vi "GOOP_GetControlRearrangement.vi"(0 "VI Refnum":refnum<vi>, 1 "_IconSize":u16(ring) caption="Icon Size" items=["Full", "1 c-term high", "2 c-term high", "3 c-term high", "4 c-term high"], 5 "error in (no error)":errorcluster, 7 "ShowIconTerminalNumbers":bool) -> (10 "StartRow":i32, 12 "EndRow":i32, 14 "ControlsToMove":T1(array[cluster]), 15 "LayoutPicture":picture, 16 "ConnectorPaneHeight":i32[](array[numeric]), 18 "NumberOfTerminalAtStart":i32, 19 "error out":errorcluster)   [LabVIEW 2020]
uses:
  <vilib>/Utility/miscctls.llb/LVRectTypeDef.ctl
  <vilib>/Analysis/baseanly.llb/Mean (DBL).vi
  <vilib>/Analysis/NI_AALBase.lvlib
  <resource>/Framework/Providers/Open_GDS/UML/Graphics_class/Graphics.lvclass
panel:
  out "Moved":cluster{"Before":i32, "After":i32}[](array[cluster])
  out "RightUpperSide":cluster{"Left":i16, "TermNo":i32, "Ctrl":bool}[](array[cluster])
  out "LeftUpperSide":cluster{"Left":i16, "TermNo":i32, "Ctrl":bool}[](array[cluster])
  out "DeleteRightSide":cluster{"Top":i16, "TermNo":i32, "Ctrl":bool}[](array[cluster])
  out "DeleteLeftSide":cluster{"Top":i16, "TermNo":i32, "Ctrl":bool}[](array[cluster])
  out "RightSide":cluster{"Top":i16, "TermNo":i32, "Ctrl":bool}[](array[cluster])
  out "LeftSide":cluster{"Top":i16, "TermNo":i32, "Ctrl":bool}[](array[cluster])
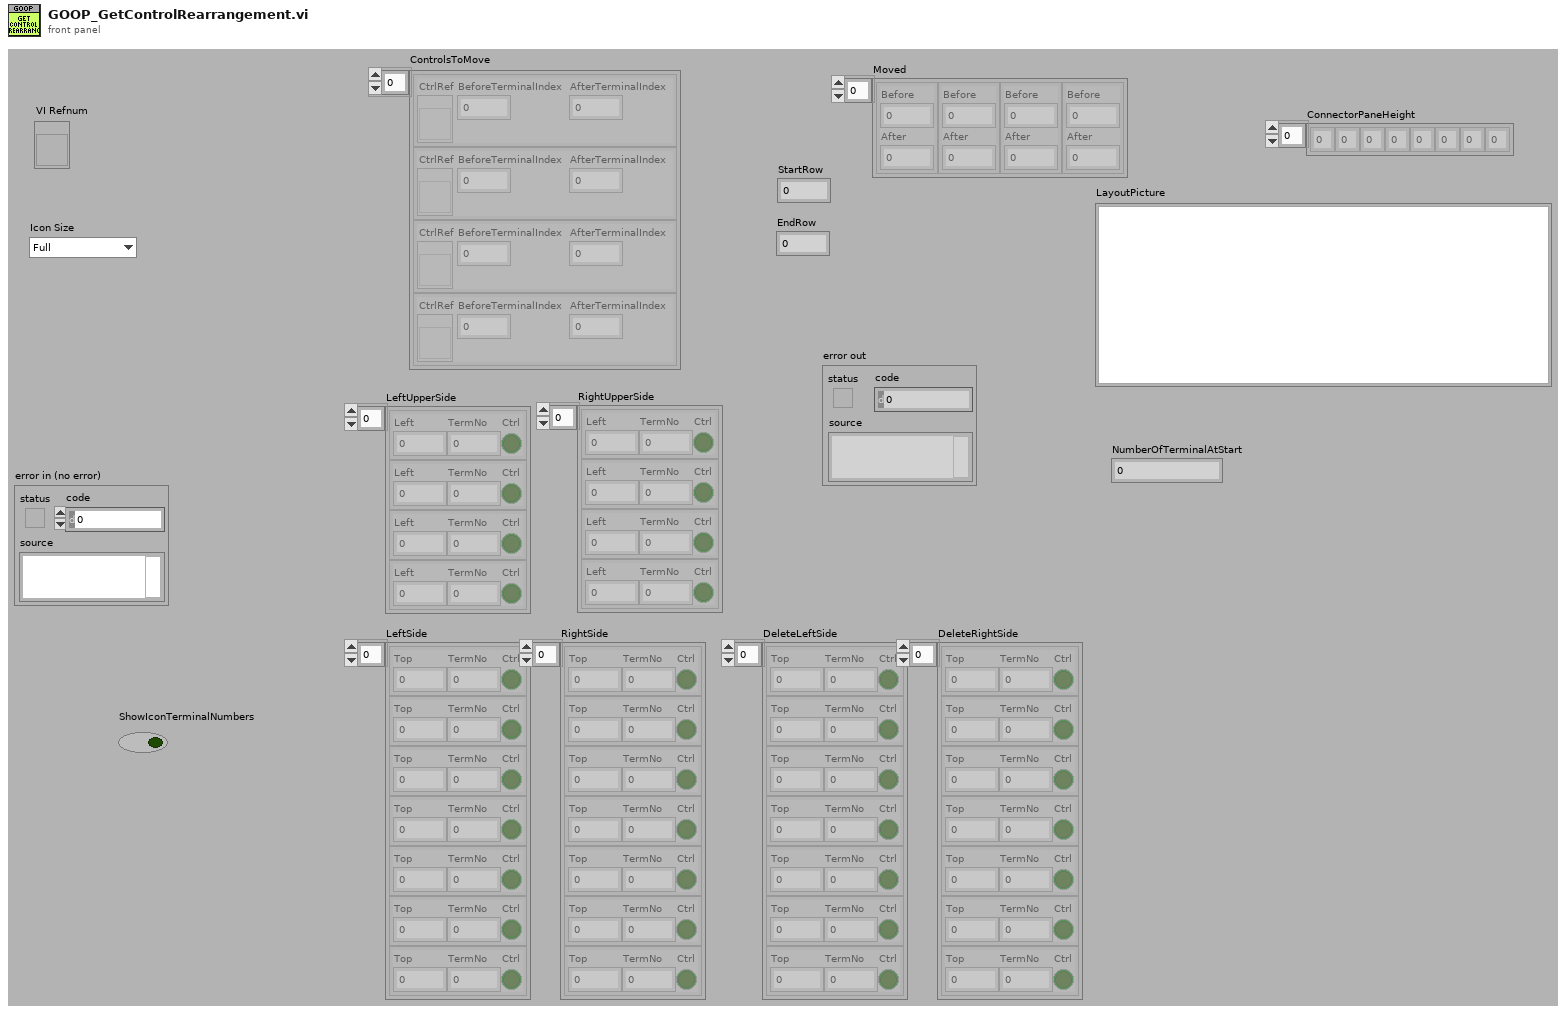
[diagram p1: front panel]
types:
  T1 = cluster{"CtrlRef":refnum<vi>, "BeforeTerminalIndex":i32, "AfterTerminalIndex":i32}[]
  T2 = typedef "LVRectTypeDef.ctl" = cluster{"Left":i16, "Top":i16, "Right":i16, "Bottom":i16}
  T3 = enum32{"invalid VI type", "Standard VI", "Control VI", "Global VI", "Polymorphic VI", "Configuration VI", "SubSystem", "Facade VI", "Method VI", "Statechart Diagram VI"}
  T4 = enum16{"Invalid Wire Rule", "Required", "Recommended", "Optional", "Dynamic Dispatch"}[]
  T5 = typedef "imagedata.ctl" = cluster{"image type":i32, "image depth":i32, "image":u8[], "mask":u8[], "colors":u32[], "Rectangle":cluster{"left":i16, "top":i16, "right":i16, "bottom":i16}}
  T6 = cluster{"horizontal":enum16{"left", "center", "right"}, "vertical":enum16{"top", "center", "bottom"}}
  T7 = enum16{"User-specified Font", "Application Font", "System Font", "Dialog Font"}
  T8 = cluster{"Font Name:":string, "Size":i16, "Strikeout?":bool, "Italic?":bool, "Underline?":bool, "Outline?":bool, "Shadow?":bool, "Bold?":bool}
  T9 = enum16{"Invalid Wire Rule", "Required", "Recommended", "Optional", "Dynamic Dispatch"}
  T10 = cluster{"CtrlRef":refnum<vi>, "BeforeTerminalIndex":i32, "AfterTerminalIndex":i32}
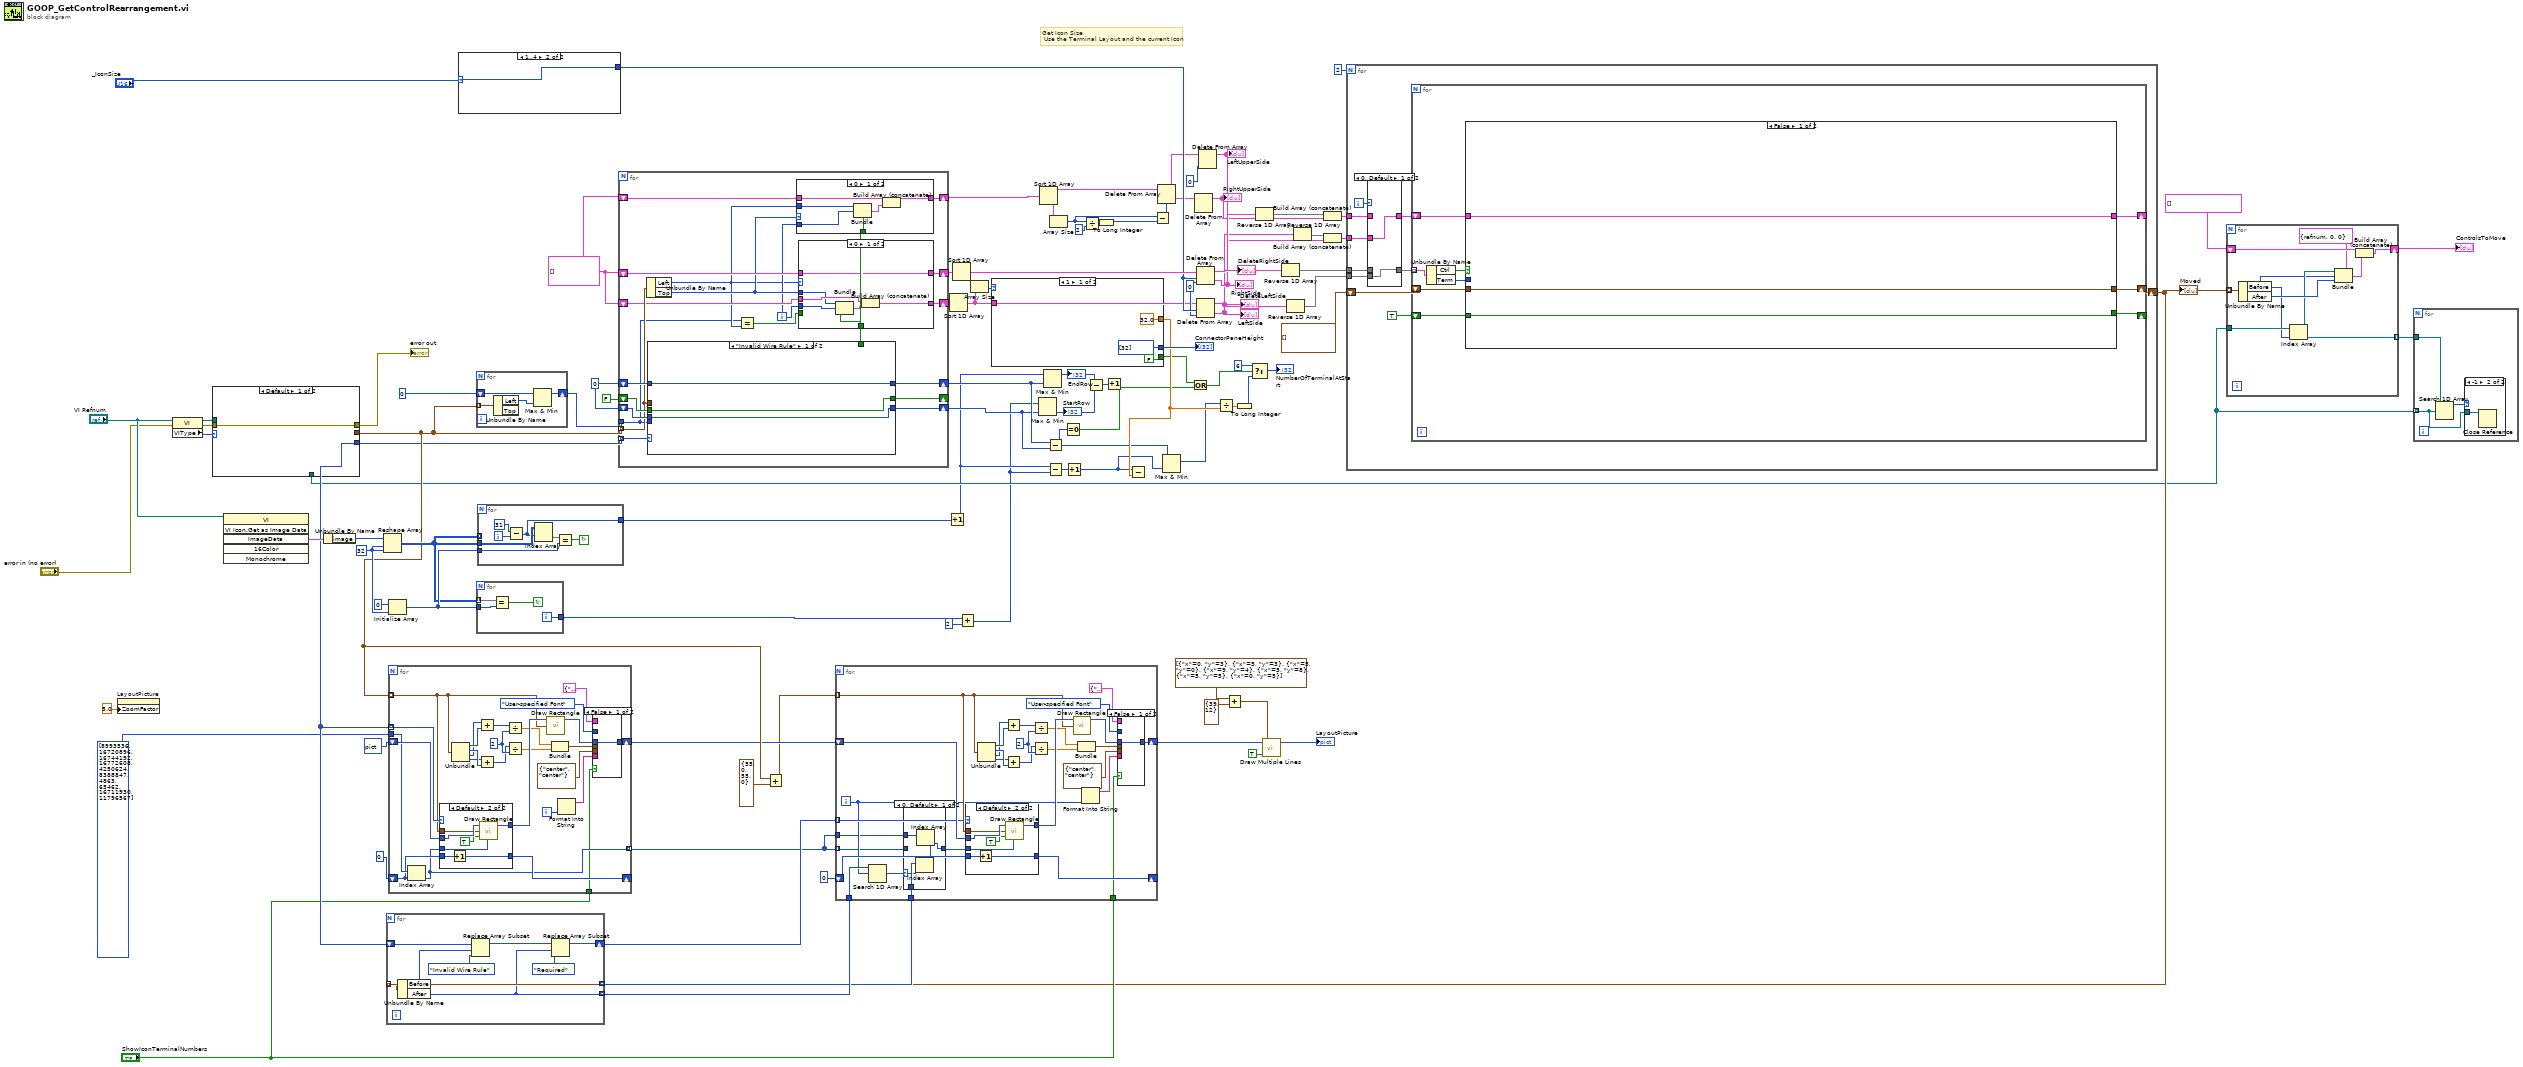
[diagram p0: block diagram]
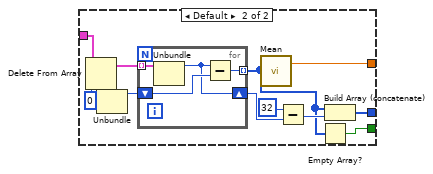
[diagram p2: hidden frame]
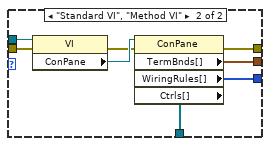
[diagram p3: hidden frame]
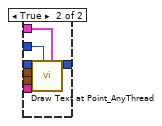
[diagram p5: hidden frame]
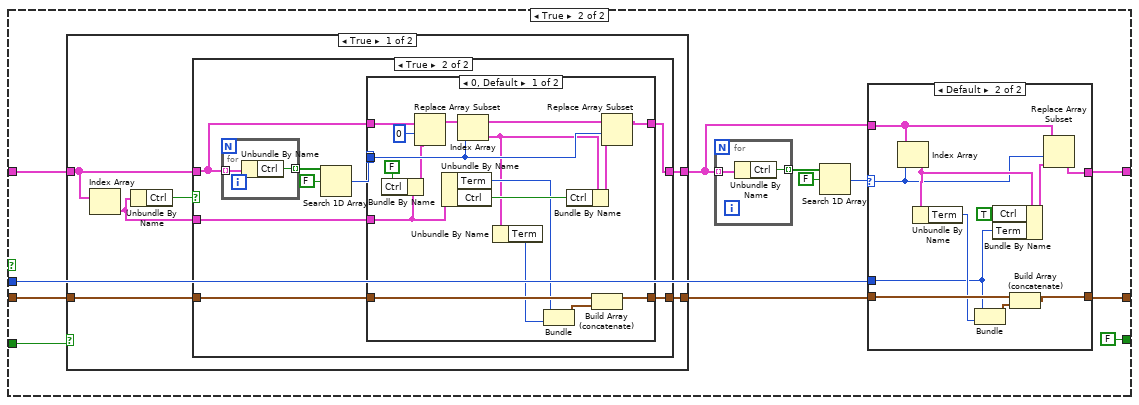
[diagram p9: hidden frame]
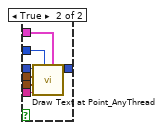
[diagram p14: hidden frame]
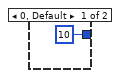
[diagram p16: hidden frame]
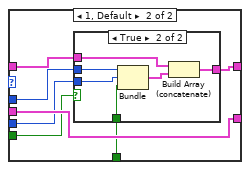
[diagram p18: hidden frame]
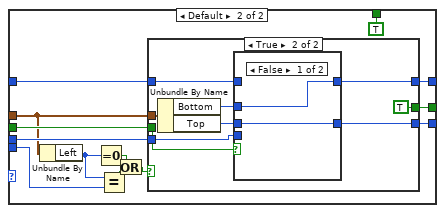
[diagram p20: hidden frame]
diagram:
  w8 = i16 0 ("bottom")
  w83 = 0 ("index")
  w90 = 32 ("dimension size")
  w82 = cluster{"top":i16, "Term":i32, "Ctrl":bool}[] []
  # "Get Icon Size\n Use the Terminal Layout and the current Icon"
  n1 = property on="LayoutPicture" class="Pict"("ZoomFactor"=sgl 5.0 ("Zoom Factor")) -> ()  [unwired: 2 in, 2 out]
  n2 = property class="VI"(reference="VI Refnum", error in="error in (no error)") -> (reference out=w24:refnum<vi>, error out=w23:errorcluster, "VIType"=w21:T3)
  n3 = case shown="Default" w21 {
    tunnel: [_ w105] -> w53
    tunnel: [_ w104] -> w50
    tunnel: [_ w103] -> w33
    tunnel: [w99 w102] -> w31
    tunnel: w24 -> [_ w101]
    tunnel: w23 -> [w99 w100]
    frame Default {
    }
    frame "Standard VI", "Method VI" {
      n4 = property class="VI"(reference=w101, error in=w100) -> (error out=w106:errorcluster, "ConPane"=w107:refnum<vi>)  [unwired: 1 out]
      n5 = property class="ConPane"(reference=w107, error in=w106) -> (error out=w102:errorcluster, "TermBnds[]"=w105:T2[], "WiringRules[]"=w104:T4, "Ctrls[]"=w103:refnum<vi>[])  [unwired: 1 out]
    }
  }
  "error out" <- w31
  n6 = invoke class="VI" method="VI Icon.Get as Image Data"(reference="VI Refnum") -> ("ImageData"=w92:T5)  [unwired: 5 in, 5 out]
  n7 = Unbundle By Name(w92) -> ("image"=w93:u8[])
  n8 = Reshape Array(w93, w90, w90) -> (w88:u8[][])
  n9 = Initialize Array(u8 0 ("element"), w90) -> (w89:u8[])
  n10 = for {
    tunnel: w53 -> [w111] mode=indexing
    shift-right: [w110] -> w52
    shift-left: picture data[5B] ("new picture") -> [w131]
    tunnel: w50 -> [w132] mode=indexing
    tunnel: u32[] [8993536, 16720896, 16744192, 16772608, 4250624, 8388847, 4863, 65462, 16711930, 11796567] -> [w129]
    shift-right: [w127] -> _
    shift-left: 0 -> [w128]
    tunnel: [w109] -> w45 mode=indexing
    tunnel: "ShowIconTerminalNumbers" -> [w108]
    i -> [w133]
    w123 = i16 2 ("y")
    n11 = Index Array(array=w129, index=w128) -> (element=w109:u32)
    n12 = case shown="Default" w132 {
      tunnel: w131 -> [w142 w148]
      tunnel: [w142 w147] -> w130
      tunnel: w111 -> [_ w146]
      tunnel: w128 -> [w143 w150]
      tunnel: [w143 w149] -> w127
      tunnel: w109 -> [_ w144]
      frame "Invalid Wire Rule" {
      }
      frame Default {
        n13 = Increment(x=w150) -> (x+1=w149:i32)
        n14 = call <vilib>:"Draw Rectangle.vi"("picture"=w148, "rect"=w146, "fill?(F)"=TRUE, "color(black)"=w144) -> ("new picture"=w147:picture)  [unwired: 5 in]
      }
    }
    n15 = Unbundle(w111) -> ("Left"=w117:i16, "Top"=w122:i16, "Right"=w116:i16, "Bottom"=w121:i16)
    n16 = Add(x=w116, y=w117) -> (x+y=w118:i16)
    n17 = Add(x=w121, y=w122) -> (x+y=w120:i16)
    n18 = Divide(x=w118, y=w123) -> (x/y=w119:dbl)
    n19 = Divide(x=w120, y=w123) -> (x/y=w124:dbl)
    n20 = call <vilib>:"Draw Rectangle.vi"("picture"=w130, "rect"=w111) -> ("new picture"=w126:picture)  [unwired: 7 in]
    n21 = Bundle(w119, w124) -> (w115:cluster{dbl, dbl})  [unwired: 1 in]
    n22 = Format Into String(w133) -> (resulting string=w125:string)  [unwired: 3 in, 1 out]
    n23 = case shown="False" w108 {
      tunnel: w126 -> [w134 w141]
      tunnel: w125 -> [_ w140]
      tunnel: w115 -> [_ w139]
      tunnel: T6 {"horizontal"=enum."center", "vertical"=enum."center"} ("alignment(left, top)") -> [_ w138]
      tunnel: T8 {"Font Name:"="Arial", "Size"=8, "Strikeout?"=FALSE, "Italic?"=FALSE, "Underline?"=FALSE, "Outline?"=FALSE, "Shadow?"=FALSE, "Bold?"=FALSE} ("[user-specified font]") -> [_ w137]
      tunnel: T7."User-specified Font" ("desired font(Application)") -> [_ w136]
      tunnel: [w134 w135] -> w110
      frame False {
      }
      frame True {
        n24 = call <resource>:"Draw Text at Point_AnyThread.vi"("[user-specified font]"=w137, "desired font(Application)"=w136, "text"=w140, "alignment(left, top)"=w138, "origin"=w139, "picture"=w141) -> ("new picture"=w135:picture)  [unwired: 4 in, 1 out]
      }
    }
  }
  n25 = case shown="1..4" "_IconSize" {
    selector: "_IconSize" -> [_ w152]
    tunnel: [10 w152] -> w84
    frame 0, Default {
    }
    frame 1..4 {
    }
  }
  n26 = for {
    tunnel: w53 -> [w156] mode=indexing
    shift-right: [w153] -> w95
    shift-left: i16 0 -> [w154]
    n27 = Unbundle By Name(w156) -> ("Left"=w155:i16)  [unwired: 1 out]
    n28 = Max & Min(x=w154, y=w155) -> (max(x,y)=w153:i16)  [unwired: 1 out]
  }
  n29 = for {
    tunnel: w88 -> [w160] mode=indexing
    tunnel: w89 -> [w159]
    tunnel: [w157] -> w20
    i -> [w157]
    stop <- w158 continue-if-true
    n30 = Equal?(x=w160, y=w159) -> (x = y?=w158:bool)
  }
  n31 = for {
    tunnel: w88 -> [_] mode=indexing
    tunnel: w89 -> [w167]
    tunnel: w88 -> [w165]
    tunnel: [w161] -> w87
    i -> [w164]
    stop <- w166 continue-if-true
    n32 = Subtract(x=31, y=w164) -> (x-y=w161:i32)
    n33 = Index Array(array=w165, index (row)=w161) -> (element=w162:u8[])  [unwired: 1 in]
    n34 = Equal?(x=w162, y=w167) -> (x = y?=w166:bool)
  }
  n35 = for {
    tunnel: w50 -> [w187] mode=indexing
    tunnel: w53 -> [w180] mode=indexing
    shift-right: [w186] -> w18
    shift-left: w8 -> [w184]
    shift-right: [w185] -> w17
    shift-left: w8 -> [w183]
    shift-right: [w181] -> _
    shift-left: FALSE -> [w182]
    shift-right: [w179] -> w97
    shift-left: w82 -> [w178]
    tunnel: w95 -> [w168]
    shift-right: [w175] -> w94
    shift-left: w82 -> [w176]
    shift-right: [w172] -> w81
    shift-left: w82 -> [w173]
    i -> [w171]
    n36 = Unbundle By Name(w180) -> ("Left"=w170:i16, "Top"=w174:i16)
    n37 = case shown="\"Invalid Wire Rule\"" w187 {
      tunnel: w180 -> [_ w224]
      tunnel: w182 -> [w216 w231]
      tunnel: [w218 w230] -> w186
      tunnel: [w217 w229] -> w185
      tunnel: w184 -> [w218 w228]
      tunnel: w183 -> [w217 w227]
      tunnel: [w216 w226] -> w181
      tunnel: [_ TRUE] -> w169
      tunnel: w168 -> [_ w222]
      frame "Invalid Wire Rule" {
      }
      frame Default {
        n38 = Unbundle By Name(w224) -> ("Left"=w223:i16)
        n39 = Equal To 0?(x=w223) -> (x = 0?=w221:bool)
        n40 = Equal?(x=w223, y=w222) -> (x = y?=w220:bool)
        n41 = Or(x=w221, y=w220) -> (x .or. y?=w219:bool)
        n42 = case shown="True" w219 {
          tunnel: w231 -> [w232 w243]
          tunnel: w224 -> [_ w242]
          tunnel: [w234 w240] -> w230
          tunnel: [w233 w239] -> w229
          tunnel: w228 -> [w234 w237]
          tunnel: w227 -> [w233 w236]
          tunnel: [w232 TRUE] -> w226
          frame False {
          }
          frame True {
            n43 = Unbundle By Name(w242) -> ("Bottom"=w241:i16, "Top"=w238:i16)
            n44 = case shown="False" w243 {
              tunnel: w241 -> [w245 w249]
              tunnel: [w245 w251] -> w240
              tunnel: [w244 w246] -> w239
              tunnel: w238 -> [w244 w247]
              tunnel: w237 -> [_ w250]
              tunnel: w236 -> [_ w248]
              frame False {
              }
              frame True {
                n45 = Max & Min(x=w250, y=w249) -> (max(x,y)=w251:i16)  [unwired: 1 out]
                n46 = Max & Min(x=w248, y=w247) -> (min(x,y)=w246:i16)  [unwired: 1 out]
              }
            }
          }
        }
      }
    }
    n47 = Equal?(x=w168, y=w170) -> (x = y?=w177:bool)
    n48 = case shown="0" w174 {
      tunnel: w173 -> [w192 w194]
      tunnel: [w191 w194] -> w172
      tunnel: w171 -> [w190 _]
      tunnel: w170 -> [w189 _]
      tunnel: w169 -> [w188 _]
      frame 0 {
        n49 = Bundle("Left"=w189, w190, w188) -> (w193:cluster{"Left":i16, i32, bool})  [unwired: 1 in]
        n50 = Build Array (concatenate)(w192, w193) -> (w191:cluster{"Left":i16, "Term":i32, "Ctrl":bool}[])
      }
      frame Default {
      }
    }
    n51 = case shown="0" w170 {
      tunnel: [w201 w208] -> w179
      tunnel: w178 -> [w200 w208]
      tunnel: w174 -> [w197 w205]
      tunnel: w177 -> [_ w207]
      tunnel: [w199 w204] -> w175
      tunnel: w176 -> [w199 w206]
      tunnel: w171 -> [w196 w203]
      tunnel: w169 -> [w195 w202]
      frame 0 {
        n52 = Bundle("Top"=w197, w196, w195) -> (w198:cluster{"Top":i16, i32, bool})  [unwired: 1 in]
        n53 = Build Array (concatenate)(w200, w198) -> (w201:cluster{"Top":i16, "Term":i32, "Ctrl":bool}[])
      }
      frame 1, Default {
        n54 = case shown="True" w207 {
          tunnel: w206 -> [w209 w215]
          tunnel: w205 -> [_ w212]
          tunnel: [w209 w214] -> w204
          tunnel: w203 -> [_ w211]
          tunnel: w202 -> [_ w210]
          frame False {
          }
          frame True {
            n55 = Bundle("Top"=w212, w211, w210) -> (w213:cluster{"Top":i16, i32, bool})  [unwired: 1 in]
            n56 = Build Array (concatenate)(w215, w213) -> (w214:cluster{"Top":i16, "Term":i32, "Ctrl":bool}[])
          }
        }
      }
    }
  }
  n57 = Add(x=w53, y=T2 {"Left"=55, "Top"=0, "Right"=55, "Bottom"=0}) -> (x+y=w51:T2[])
  n58 = Increment(x=w87) -> (x+1=w16:i32)
  n59 = Sort 1D Array(array=w97) -> (sorted array=w3:cluster{"top":i16, "Term":i32, "Ctrl":bool}[])
  n60 = Sort 1D Array(array=w94) -> (sorted array=w86:cluster{"top":i16, "Term":i32, "Ctrl":bool}[])
  n61 = Add(x=w20, y=2) -> (x+y=w15:i32)
  n62 = Array Size(array=w3) -> (size(s)=w2:i32)
  n63 = case shown="1" w2 {
    tunnel: [i16[] [32] w259] -> w26
    tunnel: [32.0 ("mean") w258] -> w13
    tunnel: [FALSE ("empty?") w256] -> w6
    tunnel: w3 -> [_ w255]
    frame 1 {
    }
    frame Default {
      n64 = Delete From Array(array=w255, index=0) -> (deleted portion=w266:cluster{"top":i16, "Term":i32, "Ctrl":bool}, array with subset deleted=w265:cluster{"top":i16, "Term":i32, "Ctrl":bool}[])  [unwired: 1 in]
      n65 = Unbundle(w266) -> ("top"=w264:i16)  [unwired: 2 out]
      n66 = for {
        tunnel: w265 -> [w270] mode=indexing
        shift-right: [w268] -> w262
        shift-left: w264 -> [w269]
        tunnel: [w267] -> w257 mode=indexing
        n67 = Unbundle(w270) -> ("top"=w268:i16)  [unwired: 2 out]
        n68 = Subtract(x=w268, y=w269) -> (x-y=w267:i16)
      }
      n69 = call-poly <vilib>:"Mean.vi"("X"=w257) -> ("mean"=w258:dbl)  [unwired: 1 out]
      n70 = Subtract(x=i16 32 ("y"), y=w262) -> (x-y=w260:i16)
      n71 = Empty Array?(array=w257) -> (empty?=w256:bool)
      n72 = Build Array (concatenate)(w257, w260) -> (w259:i16[])
    }
  }
  "ConnectorPaneHeight" <- w26
  n73 = Max & Min(x=w15, y=w17) -> (min(x,y)=w29:i32)  [unwired: 1 out]
  "StartRow" <- w29
  n74 = Sort 1D Array(array=w81) -> (sorted array=w76:cluster{"top":i16, "Term":i32, "Ctrl":bool}[])
  n75 = Max & Min(x=w16, y=w18) -> (max(x,y)=w30:i32)  [unwired: 1 out]
  "EndRow" <- w30
  n76 = Subtract(x=w18, y=w17) -> (x-y=w4:i16)
  n77 = Subtract(x=w16, y=w15) -> (x-y=w14:i32)
  n78 = Array Size(array=w76) -> (size(s)=w78:i32)
  n79 = Equal To 0?(x=w4) -> (x = 0?=w7:bool)
  n80 = Increment(x=w14) -> (x+1=w1:i32)
  n81 = Divide(x=w78, y=2) -> (x/y=w79:dbl)
  n82 = Subtract(x=w30, y=w29) -> (x-y=w28:i32)
  n83 = To Long Integer(number=w79) -> (32bit integer=w77:i32)
  n84 = Increment(x=w28) -> ()  [unwired: 1 out]
  n85 = Subtract(x=w1, y=w13) -> ()  [unwired: 1 out]
  n86 = Subtract(x=w78, y=w77) -> (x-y=w75:i32)
  n87 = Delete From Array(array=w76, length=w75) -> (deleted portion=w74:cluster{"top":i16, "Term":i32, "Ctrl":bool}[], array with subset deleted=w73:cluster{"top":i16, "Term":i32, "Ctrl":bool}[])  [unwired: 1 in]
  n88 = Max & Min(x=w4, y=w1) -> (max(x,y)=w12:i32)  [unwired: 1 out]
  n89 = Or(x=w6, y=w7) -> (x .or. y?=w5:bool)
  n90 = Delete From Array(array=w74) -> (array with subset deleted=w66:cluster{"top":i16, "Term":i32, "Ctrl":bool}[])  [unwired: 2 in, 1 out]
  "RightUpperSide" <- w66
  n91 = Delete From Array(array=w86, length=w84, index=w83) -> (deleted portion=w70:cluster{"top":i16, "Term":i32, "Ctrl":bool}[], array with subset deleted=w71:cluster{"top":i16, "Term":i32, "Ctrl":bool}[])
  "DeleteRightSide" <- w71
  "RightSide" <- w70
  n92 = Delete From Array(array=w3, length=w84, index=w83) -> (deleted portion=w60:cluster{"top":i16, "Term":i32, "Ctrl":bool}[], array with subset deleted=w56:cluster{"top":i16, "Term":i32, "Ctrl":bool}[])
  "DeleteLeftSide" <- w56
  "LeftSide" <- w60
  n93 = Delete From Array(array=w73, index=0) -> (array with subset deleted=w58:cluster{"top":i16, "Term":i32, "Ctrl":bool}[])  [unwired: 1 in, 1 out]
  "LeftUpperSide" <- w58
  n94 = Divide(x=w12, y=w13) -> (x/y=w27:dbl)
  n95 = Add(x=cluster{"x":i16, "y":i16}[] [{"x"=0, "y"=3}, {"x"=5, "y"=3}, {"x"=5, "y"=0}, {"x"=9, "y"=4}, {"x"=5, "y"=8}, {"x"=5, "y"=5}, {"x"=0, "y"=5}] ("line endpoints"), y=cluster{"x":i32, "y":i32} {"x"=39, "y"=12}) -> (x+y=w38:cluster{"x":i32, "y":i32}[])
  n96 = To Long Integer(number=w27) -> (32bit integer=w11:i32)
  n97 = Select(t=6, s=w5, f=w11) -> (s? t:f=→"NumberOfTerminalAtStart":i32)
  n98 = Reverse 1D Array(array=w70) -> (reversed array=w68:cluster{"top":i16, "Term":i32, "Ctrl":bool}[])
  n99 = Reverse 1D Array(array=w71) -> (reversed array=w62:cluster{"top":i16, "Term":i32, "Ctrl":bool}[])
  n100 = Reverse 1D Array(array=w56) -> (reversed array=w55:cluster{"top":i16, "Term":i32, "Ctrl":bool}[])
  n101 = Reverse 1D Array(array=w60) -> (reversed array=w59:cluster{"top":i16, "Term":i32, "Ctrl":bool}[])
  n102 = Build Array (concatenate)(w68, w66) -> (w67:cluster{"top":i16, "Term":i32, "Ctrl":bool}[])
  n103 = Build Array (concatenate)(w59, w58) -> (w57:cluster{"top":i16, "Term":i32, "Ctrl":bool}[])
  n104 = for {
    N: 2 -> [_]
    tunnel: w67 -> [w277]
    tunnel: w62 -> [w276]
    shift-right: [w279] -> w36
    shift-left: cluster{"Before":i32, "After":i32}[] [] -> [w280]
    tunnel: w57 -> [w273]
    tunnel: w55 -> [w272]
    i -> [w278]
    n105 = case shown="0, Default" w278 {
      tunnel: w277 -> [_ w284]
      tunnel: w276 -> [_ w283]
      tunnel: [w282 w284] -> w275
      tunnel: [w281 w283] -> w274
      tunnel: w273 -> [w282 _]
      tunnel: w272 -> [w281 _]
      frame 0, Default {
      }
      frame 1 {
      }
    }
    n106 = for {
      tunnel: w274 -> [w293] mode=indexing
      shift-right: [w287] -> _
      shift-left: w275 -> [w291]
      shift-right: [w288] -> w279
      shift-left: w280 -> [w290]
      shift-right: [w285] -> _
      shift-left: TRUE -> [w286]
      n107 = Unbundle By Name(w293) -> ("Ctrl"=w292:bool, "Term"=w289:i32)
      n108 = case shown="False" w292 {
        tunnel: w291 -> [w295 w302]
        tunnel: w290 -> [w296 w300]
        tunnel: w289 -> [_ w305]
        tunnel: [w296 w304] -> w288
        tunnel: [w295 w303] -> w287
        tunnel: w286 -> [w294 w298]
        tunnel: [w294 FALSE] -> w285
        frame False {
        }
        frame True {
          n109 = case shown="True" w298 {
            tunnel: w302 -> [w313 w346]
            tunnel: [w312 w346] -> w301
            tunnel: w300 -> [w310 w345]
            tunnel: [w309 w345] -> w299
            frame True {
              n110 = Index Array(array=w313) -> (element=w311:cluster{"top":i16, "Term":i32, "Ctrl":bool})  [unwired: 1 in]
              n111 = Unbundle By Name(w311) -> ("Ctrl"=w314:bool)
              n112 = case shown="True" w314 {
                tunnel: w313 -> [w316 w322]
                tunnel: [w316 w320] -> w312
                tunnel: w311 -> [_ w319]
                tunnel: w310 -> [w315 w317]
                tunnel: [w315 w318] -> w309
                frame False {
                }
                frame True {
                  n113 = for {
                    tunnel: w322 -> [w344] mode=indexing
                    tunnel: [w343] -> w323 mode=indexing
                    n114 = Unbundle By Name(w344) -> ("Ctrl"=w343:bool)
                  }
                  n115 = Search 1D Array(1D array=w323, element=FALSE) -> (index of element=w321:i32)  [unwired: 1 in]
                  n116 = case shown="0, Default" w321 {
                    tunnel: w322 -> [w336 w342]
                    tunnel: w321 -> [w337 _]
                    tunnel: [w340 w342] -> w320
                    tunnel: w319 -> [w333 _]
                    tunnel: [w328 w341] -> w318
                    tunnel: w317 -> [w329 w341]
                    frame 0, Default {
                      n117 = Bundle By Name(cluster=w333, "Ctrl"=FALSE ("element")) -> (w332:cluster{"top":i16, "Term":i32, "Ctrl":bool})
                      n118 = Replace Array Subset(array=w336, new element=w332, index=0) -> (w335:cluster{"top":i16, "Term":i32, "Ctrl":bool}[])
                      n119 = Unbundle By Name(w333) -> ("Term"=w327:i32, "Ctrl"=w338:bool)
                      n120 = Index Array(array=w335, index=w337) -> (element=w326:cluster{"top":i16, "Term":i32, "Ctrl":bool})
                      n121 = Unbundle By Name(w326) -> ("Term"=w325:i32)
                      n122 = Bundle("Term"=w327, "Term"=w325) -> (w330:cluster{"Term":i32, "Term":i32})  [unwired: 1 in]
                      n123 = Bundle By Name(cluster=w326, "Ctrl"=w338) -> (w339:cluster{"top":i16, "Term":i32, "Ctrl":bool})
                      n124 = Build Array (concatenate)(w329, w330) -> (w328:cluster{"Term":i32, "Term":i32}[])
                      n125 = Replace Array Subset(array=w335, new element=w339, index=w337) -> (w340:cluster{"top":i16, "Term":i32, "Ctrl":bool}[])
                    }
                    frame -1 {
                    }
                  }
                }
              }
            }
            frame False {
            }
          }
          n126 = for {
            tunnel: w301 -> [w361] mode=indexing
            tunnel: [w360] -> w308 mode=indexing
            n127 = Unbundle By Name(w361) -> ("Ctrl"=w360:bool)
          }
          n128 = Search 1D Array(1D array=w308, element=FALSE) -> (index of element=w306:i32)  [unwired: 1 in]
          n129 = case shown="Default" w306 {
            selector: w306 -> [_ w352]
            tunnel: w299 -> [w348 w359]
            tunnel: w301 -> [w347 w353]
            tunnel: w305 -> [_ w349]
            tunnel: [w348 w356] -> w304
            tunnel: [w347 w350] -> w303
            frame -1 {
            }
            frame Default {
              n130 = Index Array(array=w353, index=w352) -> (element=w355:cluster{"top":i16, "Term":i32, "Ctrl":bool})
              n131 = Unbundle By Name(w355) -> ("Term"=w357:i32)
              n132 = Bundle("Term"=w349, "Term"=w357) -> (w358:cluster{"Term":i32, "Term":i32})  [unwired: 1 in]
              n133 = Bundle By Name(cluster=w355, "Ctrl"=TRUE, "Term"=w349) -> (w351:cluster{"top":i16, "Term":i32, "Ctrl":bool})
              n134 = Build Array (concatenate)(w359, w358) -> (w356:cluster{"Term":i32, "Term":i32}[])
              n135 = Replace Array Subset(array=w353, new element=w351, index=w352) -> (w350:cluster{"top":i16, "Term":i32, "Ctrl":bool}[])
            }
          }
        }
      }
    }
  }
  "Moved" <- w36
  n136 = for {
    tunnel: w36 -> [w369] mode=indexing
    shift-right: [w365] -> w49
    shift-left: w50 -> [w368]
    tunnel: [w363] -> w46 mode=indexing
    tunnel: [w362] -> w44 mode=indexing
    n137 = Unbundle By Name(w369) -> ("Before"=w362:i32, "After"=w363:i32)
    n138 = Replace Array Subset(array=w368, new element=T9."Invalid Wire Rule" ("new element/subarray"), index=w362) -> (w366:T4)
    n139 = Replace Array Subset(array=w366, new element=T9."Required" ("new element/subarray"), index=w363) -> (w365:T4)
  }
  n140 = for {
    tunnel: w51 -> [w380] mode=indexing
    shift-right: [w379] -> w43
    shift-left: w52 -> [w399]
    shift-right: [w396] -> _
    shift-left: 0 -> [w397]
    tunnel: w49 -> [w378] mode=indexing
    tunnel: w45 -> [w374] mode=indexing
    tunnel: w46 -> [w377]
    tunnel: w45 -> [w372]
    tunnel: w44 -> [w371]
    tunnel: "ShowIconTerminalNumbers" -> [w370]
    i -> [w376]
    w392 = i16 2 ("y")
    n141 = Search 1D Array(1D array=w377, element=w376) -> (index of element=w375:i32)  [unwired: 1 in]
    n142 = case shown="0, Default" w375 {
      selector: w375 -> [w410 _]
      tunnel: w374 -> [_ w413]
      tunnel: [w408 w413] -> w373
      tunnel: w372 -> [w412 _]
      tunnel: w371 -> [w411 _]
      frame 0, Default {
        n143 = Index Array(array=w411, index=w410) -> (element=w409:i32)
        n144 = Index Array(array=w412, index=w409) -> (element=w408:u32)
      }
      frame -1 {
      }
    }
    n145 = case shown="Default" w378 {
      tunnel: w399 -> [w414 w420]
      tunnel: [w414 w419] -> w398
      tunnel: w380 -> [_ w418]
      tunnel: w397 -> [w415 w422]
      tunnel: [w415 w421] -> w396
      tunnel: w373 -> [_ w416]
      frame "Invalid Wire Rule" {
      }
      frame Default {
        n146 = Increment(x=w422) -> (x+1=w421:i32)
        n147 = call <vilib>:"Draw Rectangle.vi"("picture"=w420, "rect"=w418, "fill?(F)"=TRUE, "color(black)"=w416) -> ("new picture"=w419:picture)  [unwired: 5 in]
      }
    }
    n148 = Unbundle(w380) -> ("Left"=w386:i16, "Top"=w391:i16, "Right"=w385:i16, "Bottom"=w390:i16)
    n149 = Add(x=w385, y=w386) -> (x+y=w387:i16)
    n150 = Add(x=w390, y=w391) -> (x+y=w389:i16)
    n151 = Divide(x=w387, y=w392) -> (x/y=w388:dbl)
    n152 = Divide(x=w389, y=w392) -> (x/y=w393:dbl)
    n153 = call <vilib>:"Draw Rectangle.vi"("picture"=w398, "rect"=w380) -> ("new picture"=w395:picture)  [unwired: 7 in]
    n154 = Bundle(w388, w393) -> (w384:cluster{dbl, dbl})  [unwired: 1 in]
    n155 = Format Into String(w376) -> (resulting string=w394:string)  [unwired: 3 in, 1 out]
    n156 = case shown="False" w370 {
      tunnel: w395 -> [w400 w407]
      tunnel: w394 -> [_ w406]
      tunnel: w384 -> [_ w405]
      tunnel: T6 {"horizontal"=enum."center", "vertical"=enum."center"} ("alignment(left, top)") -> [_ w404]
      tunnel: T8 {"Font Name:"="Arial", "Size"=8, "Strikeout?"=FALSE, "Italic?"=FALSE, "Underline?"=FALSE, "Outline?"=FALSE, "Shadow?"=FALSE, "Bold?"=FALSE} ("[user-specified font]") -> [_ w403]
      tunnel: T7."User-specified Font" ("desired font(Application)") -> [_ w402]
      tunnel: [w400 w401] -> w379
      frame False {
      }
      frame True {
        n157 = call <resource>:"Draw Text at Point_AnyThread.vi"("[user-specified font]"=w403, "desired font(Application)"=w402, "text"=w406, "alignment(left, top)"=w404, "origin"=w405, "picture"=w407) -> ("new picture"=w401:picture)  [unwired: 4 in, 1 out]
      }
    }
  }
  n158 = call <vilib>:"Draw Multiple Lines.vi"("picture"=w43, "line endpoints"=w38, "fill?(F)"=TRUE) -> ("new picture"=→"LayoutPicture":picture)  [unwired: 6 in]
  n159 = for {
    tunnel: w36 -> [w431] mode=indexing
    tunnel: w33 -> [w428]
    shift-right: [w429] -> w32
    shift-left: T1 [] ("ControlsToMove") -> [w430]
    tunnel: [w425] -> w34 mode=indexing
    n160 = Unbundle By Name(w431) -> ("Before"=w423:i32, "After"=w427:i32)
    n161 = Index Array(array=w428, index=w423) -> (element=w425:refnum<vi>)
    n162 = Bundle(cluster=T10 {"CtrlRef"=refnum, "BeforeTerminalIndex"=0, "AfterTerminalIndex"=0} ("Cluster"), "CtrlRef"=w425, "BeforeTerminalIndex"=w423, "AfterTerminalIndex"=w427) -> (w426:T10)
    n163 = Build Array (concatenate)(w430, w426) -> (w429:T1)
  }
  "ControlsToMove" <- w32
  n164 = for {
    tunnel: w34 -> [w434]
    tunnel: w33 -> [w432] mode=indexing
    n165 = Search 1D Array(1D array=w434, element=w432) -> (index of element=w433:i32)  [unwired: 1 in]
    n166 = case shown="-1" w433 {
      tunnel: w432 -> [_ w435]
      frame 0, Default {
      }
      frame -1 {
        n167 = Close Reference(reference=w435) -> ()  [unwired: 1 in, 1 out]
      }
    }
  }
